vi "vision auto adjustment.vi"(0 "report":T2, 5 "restrictions":T1, 7 "Joy x_value":dbl, 9 "Joy y_value":dbl, 11 "auto_adjust":bool) -> (4 "distance":dbl, 15 "ok_to_shoot":bool)   [LabVIEW 2015]
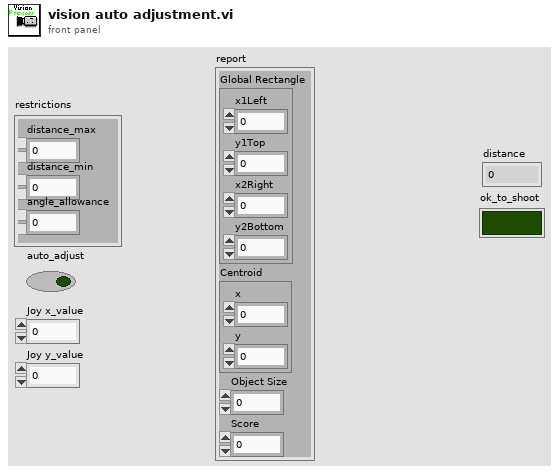
[diagram p1: front panel]
types:
  T1 = cluster{"distance_max":dbl, "distance_min":dbl, "angle_allowance":dbl}
  T2 = cluster{"Global Rectangle":cluster{"x1Left":i32, "y1Top":i32, "x2Right":i32, "y2Bottom":i32}, "Centroid":cluster{"x":sgl, "y":sgl}, "Object Size":u32, "Score":dbl}
  T3 = cluster{"x1Left":i32, "y1Top":i32, "x2Right":i32, "y2Bottom":i32}
  T4 = typedef "WPI_GyroDevRef.ctl" = cluster{"DevStatus":errorcluster, "Analog Channel":T5, "Offset":dbl, "Gain (VoltsPerDegree/Second)":dbl, "Gyro Type":enum16{"Analog", "XRS450"}, "Handle":i32, "SPI Bus":T6, "Device Found":bool, "Sample Rate":dbl, "Calibrate On Open":bool}
  T5 = typedef "FPGA_AIChannel.ctl" = enum8{"AI 0", "AI 1", "AI 2", "AI 3", "AI MXP 0", "AI MXP 1", "AI MXP 2", "AI MXP 3", "Invalid"}
  T6 = typedef "spi_bus.ctl" = enum16{"SPI On-Board, CS0", "SPI On-Board, CS1", "SPI On-Board, CS2", "SPI On-Board, CS3", "SPI MXP", "Invalid"}
  T7 = typedef "WPI_MotorControlDeviceRef.ctl" = cluster{"DeviceStatus":errorcluster, "Type":T8, "PWM":cluster{"PWM Channel":T9, "DeadBand":T10}, "CAN":cluster{"Device Number":u8, "Control Mode":T11, "Semaphore":T12, "Max Vout":dbl, "TalonSRX Control Mode":T13}, "Invert":bool}
  T8 = typedef "WPI_MotorControlType.ctl" = enum16{"PWM", "CAN", "CANTalonSRX"}
  T9 = typedef "FPGA_DIOPWMChannel.ctl" = enum8{"PWM 0", "PWM 1", "PWM 2", "PWM 3", "PWM 4", "PWM 5", "PWM 6", "PWM 7", "PWM 8", "PWM 9", "PWM MXP 0", "PWM MXP 1", "PWM MXP 2", "PWM MXP 3", "PWM MXP 4", "PWM MXP 5", "PWM MXP 6", "PWM MXP 7", "PWM MXP 8", "PWM MXP 9", "Invalid"}
  T10 = typedef "WPI_PWMDeadband.ctl" = cluster{"Name":string, "maxPositivePwm":i32, "minPositivePwm":i32, "centerPwm":i32, "maxNegativePwm":i32, "minNegativePwm":i32, "angularRange":u16}
  T11 = typedef "WPI_CANJaguar_ControlMode.ctl" = enum8{"Percent VBus", "Current", "Speed", "Position", "Voltage"}
  T12 = typedef "Semaphore RefNum" = refnum<k1>
  T13 = typedef "WPI_CANTalonSRX_APIControlMode.ctl" = enum8{"Percent VBus", "Speed", "Position", "Slave", "Unchanged / Invalid", "Voltage Compensation", "Current", "Motion Profile"}
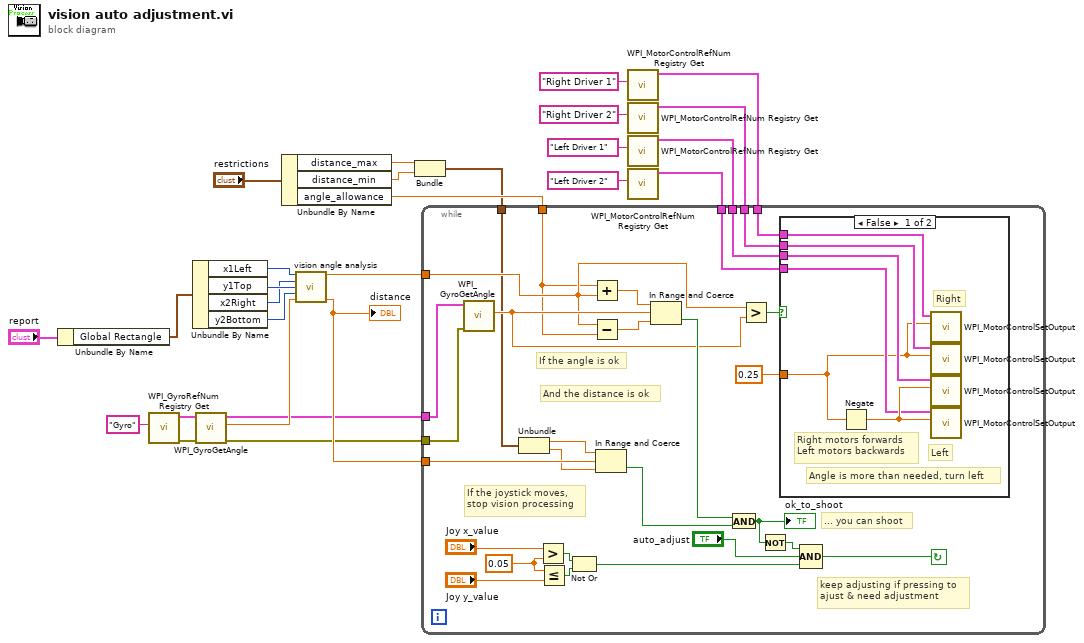
[diagram p0: block diagram]
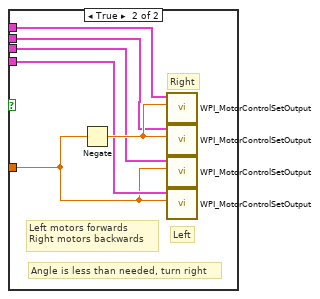
[diagram p2: hidden frame]
diagram:
  n1 = Unbundle By Name("report") -> ("Global Rectangle"=w26:T3)
  n2 = call <vilib>:"WPI_GyroRefNum Registry Get.vi"("refnum name"="Gyro") -> ("error out"=w19:errorcluster, "GyroDevRef"=w20:T4)  [unwired: 9 in]
  n3 = Unbundle By Name(w26) -> ("x1Left"=w22:i32, "y1Top"=w24:i32, "x2Right"=w23:i32, "y2Bottom"=w25:i32)
  n4 = call <vilib>:"WPI_GyroGetAngle.vi"("error in (no error)"=w19, "GyroDevRef"=w20) -> ("error out"=w14:errorcluster, "Angle"=w21:dbl, "GyroDevRef"=w15:T4)  [unwired: 6 in, 1 out]
  n5 = Unbundle By Name("restrictions") -> ("distance_max"=w10:dbl, "distance_min"=w11:dbl, "angle_allowance"=w12:dbl)
  n6 = call "vision angle analysis.vi"("left_x"=w22, "right_x"=w23, "top_y"=w24, "bottom_y"=w25, "gyro_angle_deg"=w21) -> ("gyro_heading_deg"=w17:dbl, "distance"=w16:dbl)  [unwired: 9 in]
  "distance" <- w16
  n7 = Bundle("distance_max"=w10, "distance_min"=w11) -> (w9:cluster{"distance_max":dbl, "distance_min":dbl})  [unwired: 1 in]
  n8 = call <vilib>:"WPI_MotorControlRefNum Registry Get.vi"("refnum name"="Right Driver 1") -> ("MotorControlDevRef"=w8:T7)  [unwired: 9 in, 1 out]
  n9 = call <vilib>:"WPI_MotorControlRefNum Registry Get.vi"("refnum name"="Right Driver 2") -> ("MotorControlDevRef"=w7:T7)  [unwired: 9 in, 1 out]
  n10 = call <vilib>:"WPI_MotorControlRefNum Registry Get.vi"("refnum name"="Left Driver 1") -> ("MotorControlDevRef"=w6:T7)  [unwired: 9 in, 1 out]
  n11 = call <vilib>:"WPI_MotorControlRefNum Registry Get.vi"("refnum name"="Left Driver 2") -> ("MotorControlDevRef"=w5:T7)  [unwired: 9 in, 1 out]
  n12 = while {
    tunnel: w17 -> [w43]
    tunnel: w16 -> [w56]
    tunnel: w15 -> [w47]
    tunnel: w14 -> [w46]
    tunnel: w12 -> [w42]
    tunnel: w9 -> [w41]
    tunnel: w8 -> [w32]
    tunnel: w7 -> [w31]
    tunnel: w6 -> [w30]
    tunnel: w5 -> [w29]
    stop <- w51 continue-if-true
    w36 = 0.05
    # "If the joystick moves,\nstop vision processing"
    # "keep adjusting if pressing to\najust & need adjustment"
    # "... you can shoot"
    # "And the distance is ok"
    # "If the angle is ok"
    n13 = call <vilib>:"WPI_GyroGetAngle.vi"("error in (no error)"=w46, "GyroDevRef"=w47) -> ("Angle"=w44:dbl)  [unwired: 6 in, 3 out]
    n14 = Unbundle(w41) -> ("distance_max"=w39:dbl, "distance_min"=w40:dbl)
    n15 = Greater?(x="Joy x_value", y=w36) -> (0:w35:bool)
    n16 = Less Or Equal?(x=w36, y="Joy y_value") -> (x <= y?=w34:bool)
    n17 = Not Or(1:w34, 2:w35) -> (0:w33:bool)
    n18 = Add(x=w42, y=w43) -> (x+y=w50:dbl)
    n19 = Subtract(x=w43, y=w42) -> (x-y=w49:dbl)
    n20 = In Range and Coerce(upper limit=w39, x=w56, lower limit=w40) -> (In Range?=w55:bool)  [unwired: 1 out]
    n21 = In Range and Coerce(upper limit=w50, x=w44, lower limit=w49) -> (In Range?=w48:bool)  [unwired: 1 out]
    n22 = And(x=w48, y=w55) -> (x .and. y?=w52:bool)
    "ok_to_shoot" <- w52
    n23 = Greater?(x=w43, y=w44) -> (0:w45:bool)
    n24 = Not(x=w52) -> (.not. x?=w53:bool)
    n25 = case shown="False" w45 {
      tunnel: w32 -> [w61 w67]
      tunnel: w31 -> [w60 w66]
      tunnel: w30 -> [w59 w65]
      tunnel: w29 -> [w58 w64]
      tunnel: 0.25 -> [w57 w63]
      frame False {
        # "Left"
        # "Right"
        # "Angle is more than needed, turn left"
        # "Right motors forwards\nLeft motors backwards"
        n26 = Negate(x=w57) -> (-x=w62:dbl)
        n27 = call <vilib>:"WPI_MotorControlSetOutput.vi"("Output"=w57, "MotorControlDevRef"=w61) -> ()  [unwired: 7 in, 3 out]
        n28 = call <vilib>:"WPI_MotorControlSetOutput.vi"("Output"=w57, "MotorControlDevRef"=w60) -> ()  [unwired: 7 in, 3 out]
        n29 = call <vilib>:"WPI_MotorControlSetOutput.vi"("Output"=w62, "MotorControlDevRef"=w59) -> ()  [unwired: 7 in, 3 out]
        n30 = call <vilib>:"WPI_MotorControlSetOutput.vi"("Output"=w62, "MotorControlDevRef"=w58) -> ()  [unwired: 7 in, 3 out]
      }
      frame True {
        # "Right"
        # "Left"
        # "Angle is less than needed, turn right"
        # "Left motors forwards\nRight motors backwards"
        n31 = Negate(x=w63) -> (-x=w68:dbl)
        n32 = call <vilib>:"WPI_MotorControlSetOutput.vi"("Output"=w68, "MotorControlDevRef"=w67) -> ()  [unwired: 7 in, 3 out]
        n33 = call <vilib>:"WPI_MotorControlSetOutput.vi"("Output"=w68, "MotorControlDevRef"=w66) -> ()  [unwired: 7 in, 3 out]
        n34 = call <vilib>:"WPI_MotorControlSetOutput.vi"("Output"=w63, "MotorControlDevRef"=w65) -> ()  [unwired: 7 in, 3 out]
        n35 = call <vilib>:"WPI_MotorControlSetOutput.vi"("Output"=w63, "MotorControlDevRef"=w64) -> ()  [unwired: 7 in, 3 out]
      }
    }
    n36 = Compound Arithmetic op=AND(w53, "auto_adjust", w33) -> (w51:bool)
  }
